vi "Set IC.vi"(8 "error in (no error)":errorcluster, 10 "IC":variant, 11 "IC_2D_Numeric in":refnum<class "NI_IC_2D_Numeric.lvclass">) -> (0 "error out":errorcluster, 3 "IC_2D_Numeric out":refnum<class "NI_IC_2D_Numeric.lvclass">)   [LabVIEW 2017, in "NI_PDE.lvlib" / "NI_IC_2D_Numeric.lvclass"]
uses:
  <vilib>/gmath/pde.llb/ICClass/IC_2D_Numeric/NI_IC_2D_Numeric.lvclass
  <vilib>/gmath/pde.llb/ICClass/IC_2D_Numeric/IC Data.ctl
  <vilib>/gmath/pde.llb/Common/PDE_IC Type.ctl
  <vilib>/gmath/pde.llb/ICClass/IC_2D_Numeric/NI_IC_2D_Numeric.lvclass/NI_IC_2D_Numeric.ctl
  <vilib>/gmath/NI_PDE.lvlib
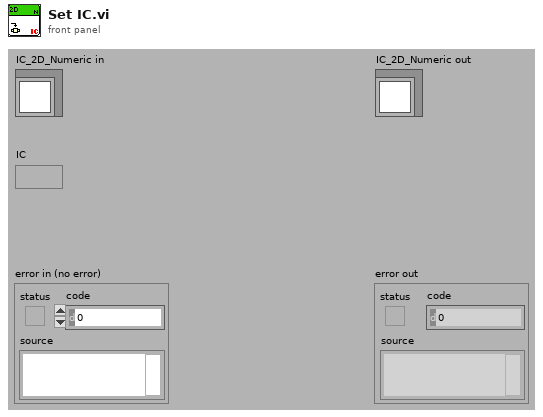
[diagram p1: front panel]
types:
  T1 = typedef "NI_PDE.lvlib/NI_IC_2D_Numeric.lvclass/IC Data.ctl" = cluster{"type":T2, "H":dbl[][]}
  T2 = typedef "NI_PDE.lvlib/PDE_IC Type.ctl" = i32
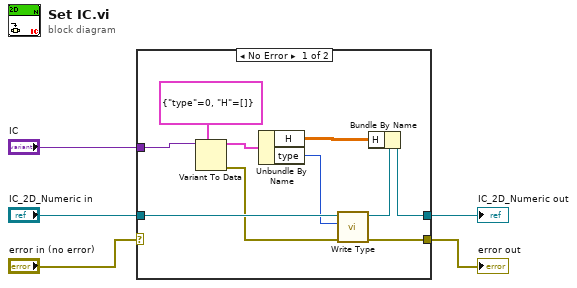
[diagram p0: block diagram]
diagram:
  n1 = case shown="No Error" "error in (no error)" {
    selector: "error in (no error)" -> [_ w17]
    tunnel: "IC_2D_Numeric in" -> [w13 w16]
    tunnel: [w9 w16] -> w5
    tunnel: [w8 w17] -> w4
    tunnel: "IC" -> [w14 _]
    frame No Error {
      n2 = Variant To Data(type=T1 {"type"=0, "H"=[]} ("IC data"), Variant=w14) -> (data=w12:T1, error out=w11:errorcluster)  [unwired: 1 in]
      n3 = Unbundle By Name(w12) -> ("H"=w7:dbl[][], "type"=w6:T2)
      n4 = call-dynamic "Write Type.vi"("error in (no error)"=w11, "IC type"=w6, "IC.lvclass in"=w13) -> ("error out"=w8:errorcluster, "IC.lvclass out"=w10:refnum<class "NI_IC_2D_Numeric.lvclass">)  [unwired: 7 out]
      n5 = Bundle By Name(cluster=w10, "H"=w7) -> (w9:refnum<class "NI_IC_2D_Numeric.lvclass">)
    }
    frame Error {
    }
  }
  "IC_2D_Numeric out" <- w5
  "error out" <- w4
